vi "Write Icon Data to Library.vi"(8 "error in":errorcluster, 10 "Data":string, 11 "Library Ref in":refnum<vi>) -> (0 "error out":errorcluster, 3 "Library Ref out":refnum<vi>)   [LabVIEW 2020, in "lv_icon.lvlib"]
doc: "Set the LabVIEW Icon Data of a Library."
uses:
  resource/plugins/lv_icon.lvlib
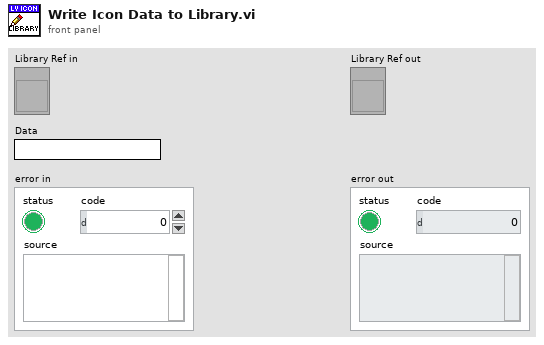
[diagram p1: front panel]
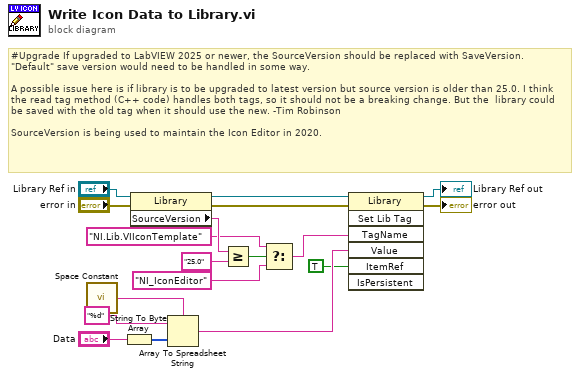
[diagram p0: block diagram]
diagram:
  # "#Upgrade If upgraded to LabVIEW 2025 or newer, the SourceVersion should be replaced with SaveVersion.\n\"Default\" save version would need to be handled in some way.\n\nA possible issue here is if library is to be upgraded to latest version but source version is older than 25.0. I think the read tag method (C++ code) handles both tags, so it should not be a breaking change. But the  library could be saved with the old tag when it should use the new. -Tim Robinson\n\nSourceVersion is being used to maintain the Icon Editor in 2020."
  n1 = call <vilib>:"Space Constant.vi"() -> ("String"=w11:string)
  n2 = String To Byte Array(string="Data") -> (unsigned byte array=w14:u8[])
  n3 = property class="Library"(reference="Library Ref in", error in="error in") -> (reference out=w8:refnum<vi>, error out=w16:errorcluster, "SourceVersion"=w7:string)
  n4 = Array To Spreadsheet String(delimiter (Tab)=w11, array=w14, 3:"%d" ("format string")) -> (spreadsheet string=w12:string)
  n5 = Greater Or Equal?(x=w7, y="25.0") -> (x >= y?=w5:bool)
  n6 = Select(t="NI.Lib.VIIconTemplate", s=w5, f="NI_IconEditor" ("Tag Name")) -> (s? t:f=w2:string)
  n7 = invoke class="Library" method="Set Lib Tag"(reference=w8, error in=w16, "TagName"=w2, "Value"=w12, "ItemRef"=TRUE ("Is Persistent")) -> (reference out=→"Library Ref out":refnum<vi>, error out=→"error out":errorcluster)  [unwired: 2 in, 5 out]
